vi "AAP.vi"(0 "System no.":i32=1 min=1 step=1, 1 "Board":i32=1 min=1 max=5 step=1, 2 "Axis 1 to scan":string, 3 "Axis 2 to scan":string, 4 "Range axis 1":dbl=0.1 format="%.4f", 5 "error in":errorcluster, 7 "Step size":dbl=0.001 format="%.4f", 8 "Repeat pos.":i32=3, 9 "Range axis 2":dbl=0.1 format="%.4f", 10 "Use #7 polling?":bool, 11 "Timeout (s)":dbl=60.0 min=1.0 max=4.0 step=1.0 format="%.2f", 12 "Stop refnum":refnum<vi>) -> (14 "Scan successful?":bool, 19 "error out":errorcluster)   [LabVIEW 2020]
doc: "Performs a fast automated alignment in specified axes, waits until scan is finished using #7 polling (if checked) and indicates whether scan was successful or not. Timeout is only valid if Use #7 polling is FALSE. If Refnum stop or Local stop is TRUE, VI sends #24 and stops. \n\nC-887, F-206, M-8X0: Use #7 polling = FALSE, Range axis 2 must be identical with Range axis 1 (no rectangular scan implemented). For GCS syntax version = GCS 2.0 or higher (check with CSV?.vi. If CSV?.vi is not supported, syntax version is GCS 1.0), VI calls FSS? automatically to determine if scan was successful or not."
uses:
  Syntax.ctl
  Global1.vi
panel:
  in  "Local stop":bool
  # "Performs a fast automated alignment in specified axes, waits until scan is \nfinished (using #7 polling if checked) and indicates whether scan was \nsuccessful or not. \"Timeout\" is only valid if \"Use #7 polling\" is FALSE. If Stop \nrefnum or Local stop is TRUE, VI sends #24 and stops."
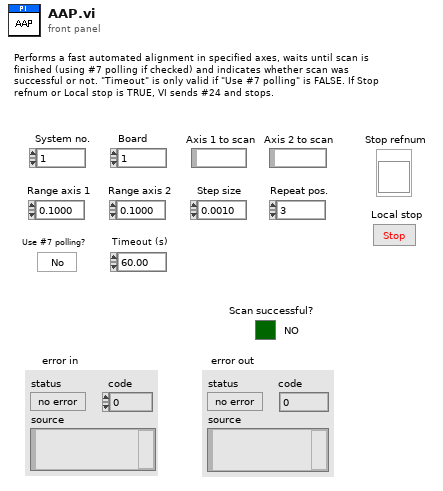
[diagram p1: front panel]
types:
  T1 = typedef "Syntax.ctl" = enum16{"GCS 1.0", "GCS 2.0", "GCS 3.0"}
  T2 = enum16{"Disable error check", "Force error check", "Use global settings"}
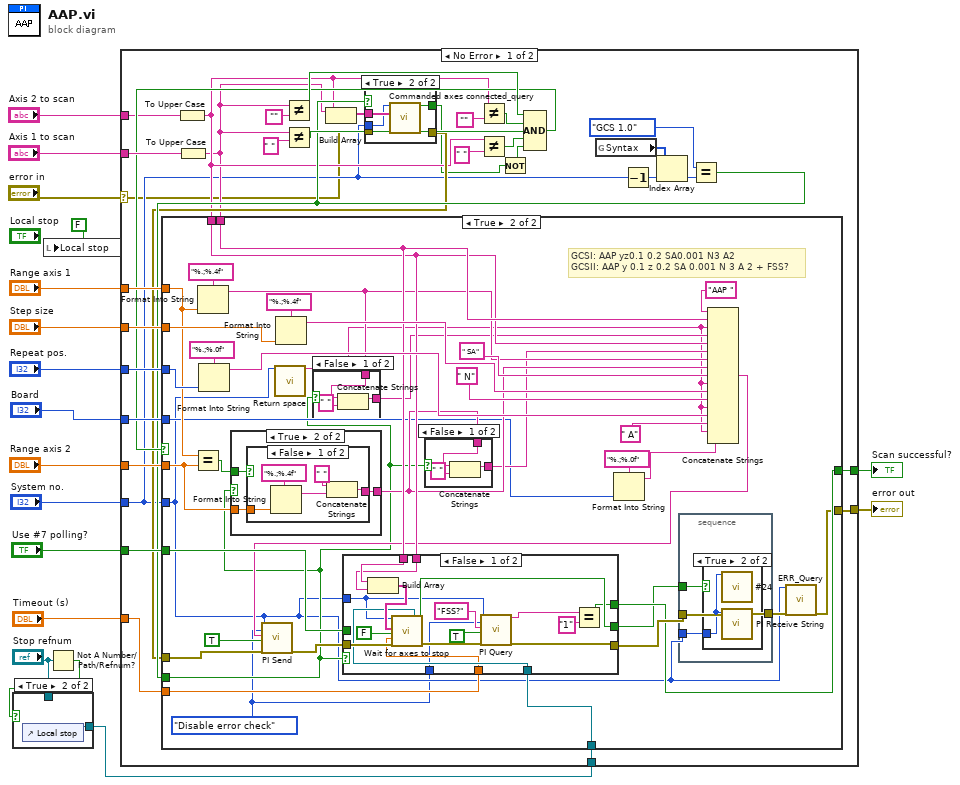
[diagram p0: block diagram]
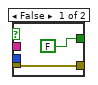
[diagram p3: hidden frame]
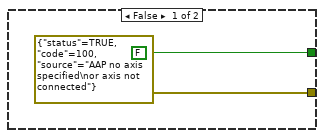
[diagram p4: hidden frame]
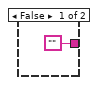
[diagram p5: hidden frame]
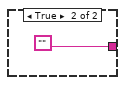
[diagram p6: hidden frame]
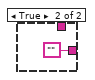
[diagram p7: hidden frame]
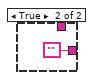
[diagram p8: hidden frame]
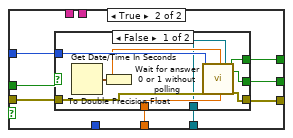
[diagram p9: hidden frame]
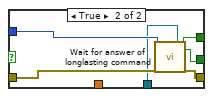
[diagram p10: hidden frame]
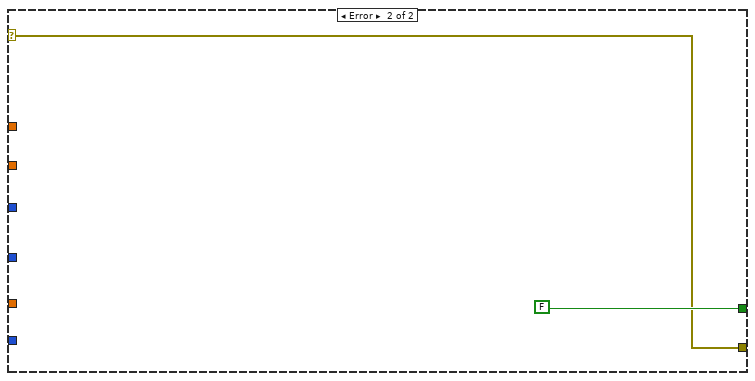
[diagram p12: hidden frame]
diagram:
  n1 = local write "Local stop"(FALSE ("Local stop")) -> ()
  n2 = Not A Number/Path/Refnum?(number/path/refnum="Stop refnum") -> (NaN/Path/Refnum?=w4:bool)
  n3 = case shown="True" w4 {
    tunnel: [w18 w19] -> w2
    tunnel: "Stop refnum" -> [w18 _]
    frame False {
    }
    frame True {
      n4 = control-ref of="Local stop"() -> (w19:refnum<vi>)
    }
  }
  n5 = case shown="No Error" "error in" {
    selector: "error in" -> [w21 w164]
    tunnel: "System no." -> [w24 _]
    tunnel: [w44 w164] -> w16
    tunnel: "Axis 1 to scan" -> [w53 _]
    tunnel: [w43 FALSE] -> w14
    tunnel: "Board" -> [w49 _]
    tunnel: "Range axis 1" -> [w48 _]
    tunnel: "Step size" -> [w47 _]
    tunnel: "Repeat pos." -> [w46 _]
    tunnel: "Axis 2 to scan" -> [w41 _]
    tunnel: "Use #7 polling?" -> [w36 _]
    tunnel: "Timeout (s)" -> [w35 _]
    tunnel: "Range axis 2" -> [w34 _]
    tunnel: w2 -> [w33 _]
    frame No Error {
      n6 = To Upper Case(1:w41) -> (0:w26:string)
      n7 = To Upper Case(1:w53) -> (0:w25:string)
      n8 = Not Equal?(x=w25, y="") -> (x != y?=w50:bool)
      n9 = Not Equal?(x=w25, y=" ") -> (x != y?=w39:bool)
      n10 = Build Array(w25, w26) -> (w27:string[])
      n11 = Not Equal?(x=w26, y="") -> (x != y?=w38:bool)
      n12 = Not Equal?(x=w26, y=" ") -> (x != y?=w37:bool)
      n13 = global read "Global1.vi" "Syntax"() -> (w32:T1[])
      n14 = Decrement(x=w24) -> (x-1=w31:i32)
      n15 = Index Array(array=w32, index=w31) -> (element=w30:T1)
      n16 = Equal?(x=Syntax."GCS 1.0" ("y"), y=w30) -> (x = y?=w29:bool)
      n17 = case shown="True" w29 {
        tunnel: w27 -> [_ w60]
        tunnel: w21 -> [w54 w59]
        tunnel: [w54 w58] -> w28
        tunnel: [FALSE ("Controller error") w57] -> w22
        tunnel: w24 -> [_ w56]
        frame False {
        }
        frame True {
          n18 = call "Commanded axes connected_query.vi"("System no."=w56, "Commanded axes"=w60, "error in"=w59) -> ("Controller error"=w57:bool, "error out"=w58:errorcluster)  [unwired: 15 out]
        }
      }
      n19 = Not(x=w22) -> (.not. x?=w23:bool)
      n20 = Compound Arithmetic op=AND(w50, w38, w39, w37, w23) -> (w45:bool)
      n21 = case shown="True" w45 {
        tunnel: w49 -> [_ w69]
        tunnel: w48 -> [_ w90]
        tunnel: w47 -> [_ w95]
        tunnel: w25 -> [_ w79]
        tunnel: w46 -> [_ w97]
        tunnel: w28 -> [_ w101]
        tunnel: w24 -> [_ w64]
        tunnel: [errorcluster {"status"=TRUE, "code"=100, "source"="AAP no axis specified\nor axis not connected"} ("error out") w65] -> w44
        tunnel: [FALSE w84] -> w43
        tunnel: w26 -> [_ w78]
        tunnel: w36 -> [_ w94]
        tunnel: w35 -> [_ w93]
        tunnel: w34 -> [_ w89]
        tunnel: w33 -> [_ w83]
        tunnel: w29 -> [_ w67]
        frame False {
        }
        frame True {
          w63 = T2."Disable error check" ("Error check settings")
          # "GCSI: AAP yz0.1 0.2 SA0.001 N3 A2\nGCSII: AAP y 0.1 z 0.2 SA 0.001 N 3 A 2 + FSS?"
          n22 = Equal?(x=w90, y=w89) -> (x = y?=w88:bool)
          n23 = Format Into String(format string="%.;%.4f" ("Format String"), w90) -> (resulting string=w77:string)  [unwired: 2 in, 1 out]
          n24 = Format Into String(format string="%.;%.0f" ("Format String"), w97) -> (resulting string=w86:string)  [unwired: 2 in, 1 out]
          n25 = case shown="True" w67 {
            tunnel: w89 -> [_ w105]
            tunnel: w88 -> [_ w104]
            tunnel: ["" w103] -> w75
            frame False {
            }
            frame True {
              n26 = case shown="False" w104 {
                tunnel: w105 -> [w109 _]
                tunnel: [w106 ""] -> w103
                frame False {
                  n27 = Format Into String(format string="%.;%.4f" ("Format String"), w109) -> (resulting string=w107:string)  [unwired: 2 in, 1 out]
                  n28 = Concatenate Strings(" ", w107) -> (w106:string)
                }
                frame True {
                }
              }
            }
          }
          n29 = call "Return space.vi"("System no."=w64) -> ("String out"=w72:string)  [unwired: 1 in, 17 out]
          n30 = Format Into String(format string="%.;%.4f" ("Format String"), w95) -> (resulting string=w92:string)  [unwired: 2 in, 1 out]
          n31 = case shown="False" w67 {
            tunnel: [w118 ""] -> w76
            tunnel: w77 -> [w117 _]
            frame False {
              n32 = Concatenate Strings(w117, " ") -> (w118:string)
            }
            frame True {
            }
          }
          n33 = case shown="False" w67 {
            tunnel: [w114 ""] -> w74
            tunnel: w75 -> [w113 _]
            frame False {
              n34 = Concatenate Strings(w113, " ") -> (w114:string)
            }
            frame True {
            }
          }
          n35 = Format Into String(format string="%.;%.0f" ("Format String"), w69) -> (resulting string=w70:string)  [unwired: 2 in, 1 out]
          n36 = Concatenate Strings("AAP ", w79, w72, w76, w78, w74, w77, w75, " SA", w72, w92, " N", w72, w86, " A", w72, w70) -> (w68:string)
          n37 = call "PI Send.vi"("System no."=w64, "Error check settings"=w63, "String to send"=w68, "Attach termination char.?"=TRUE ("Attach Linefeed?"), "error in"=w101) -> ("error out"=w80:errorcluster)  [unwired: 1 in, 13 out]
          n38 = case shown="False" w67 {
            tunnel: w94 -> [_ w144]
            tunnel: w93 -> [w123 w143]
            tunnel: [w121 w142] -> w85
            tunnel: [w124 w141] -> w84
            tunnel: w83 -> [w131 w140]
            tunnel: [w130 w139] -> w82
            tunnel: w64 -> [w126 w138]
            tunnel: w80 -> [w135 w137]
            tunnel: w79 -> [w133 _]
            tunnel: w78 -> [w132 _]
            tunnel: w63 -> [w120 _]
            frame False {
              n39 = Build Array(w133, w132) -> (w134:string[])
              n40 = call "Wait for axes to stop.vi"("System no."=w126, "Axes to wait for"=w134, "With status bit polling?"=FALSE, "Timeout (s)"=w123, "error in"=w135, "Stop refnum"=w131) -> ("Stopped"=w130:bool, "error out"=w127:errorcluster)  [unwired: 1 in, 11 out]
              n41 = call "PI Query.vi"("System no."=w126, "Error check settings"=w120, "String to send"="FSS?", "Attach termination char.?"=TRUE ("Attach Linefeed?"), "error in"=w127) -> ("String read"=w122:string, "error out"=w121:errorcluster)  [unwired: 2 in, 11 out]
              n42 = Equal?(x=w122, y="1") -> (x = y?=w124:bool)
            }
            frame True {
              n43 = case shown="False" w144 {
                tunnel: w138 -> [w153 w159]
                tunnel: w137 -> [w152 w158]
                tunnel: [w151 w157] -> w142
                tunnel: [w150 w156] -> w141
                tunnel: w143 -> [w148 _]
                tunnel: w140 -> [w147 w155]
                tunnel: [w146 w154] -> w139
                frame False {
                  n44 = Get Date/Time In Seconds() -> (seconds since 1Jan1904=w145:timestamp)
                  n45 = To Double Precision Float(number=w145) -> (double precision float=w149:dbl)
                  n46 = call "Wait for answer 0 or 1 without polling.vi"("System no."=w153, "error in"=w152, "Start time"=w149, "Timeout (s)"=w148, "Stop refnum"=w147) -> ("Scan successful?"=w150:bool, "Stopped"=w146:bool, "error out"=w151:errorcluster)  [unwired: 12 out]
                }
                frame True {
                  n47 = call "Wait for answer of longlasting command.vi"("System no."=w159, "error in"=w158, "Stop refnum"=w155) -> ("Answer"=w156:bool, "Stopped"=w154:bool, "error out"=w157:errorcluster)  [unwired: 14 out]
                }
              }
            }
          }
          n48 = stacked-sequence {
            tunnel: w64 -> [w162]
            tunnel: w85 -> [w161]
            tunnel: [w161] -> w66
            tunnel: w82 -> [w160]
            frame #0 {
              n49 = case shown="True" w160 {
                tunnel: w162 -> [_ w163]
                frame False {
                }
                frame True {
                  n50 = call "#24.vi"("System no."=w163) -> ()  [unwired: 1 in, 18 out]
                  n51 = call "PI Receive String.vi"("System no."=w163) -> ()  [unwired: 2 in, 17 out]
                }
              }
            }
          }
          n52 = call "ERR_Query.vi"("System no."=w64, "error in"=w66) -> ("error out"=w65:errorcluster)  [unwired: 17 out]
        }
      }
    }
    frame Error {
    }
  }
  "error out" <- w16
  "Scan successful?" <- w14
